vi "Get PI data.vi"() -> ()   [LabVIEW 2017]
panel:
  out "values":T1
  out "error out":errorcluster
  in  "connection ID":refnum<k16>
  in  "error in (no error)":errorcluster
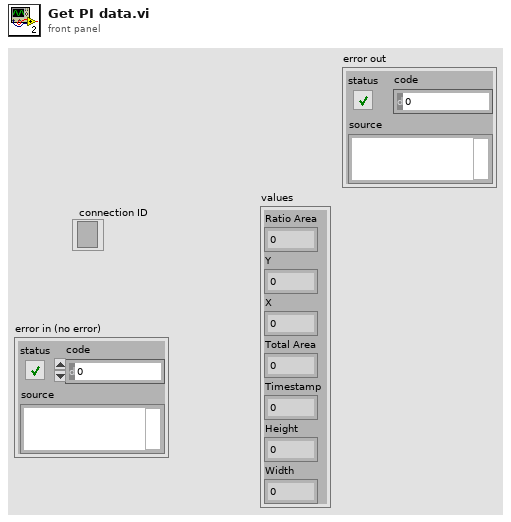
[diagram p1: front panel]
types:
  T1 = cluster{"Ratio Area":dbl, "Y":dbl, "X":dbl, "Total Area":dbl, "Timestamp":ext, "Height":dbl, "Width":dbl}
  T2 = cluster{"RatioArea":dbl, "CenterY":dbl, "CenterX":dbl, "Area":dbl, "Timestamp":ext, "Height":dbl, "Width":dbl}
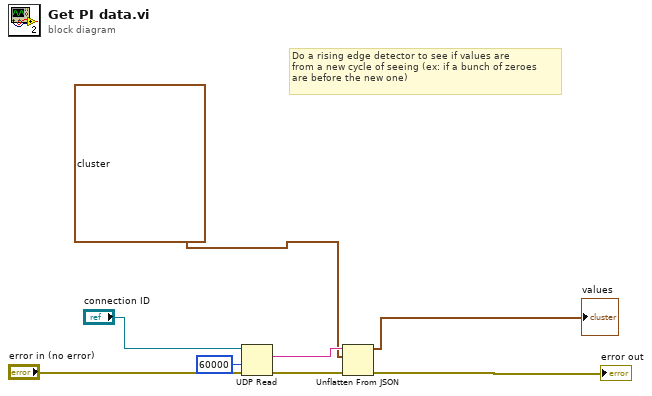
[diagram p0: block diagram]
diagram:
  # "Do a rising edge detector to see if values are \nfrom a new cycle of seeing (ex: if a bunch of zeroes\nare before the new one)"
  n1 = UDP Read(connection ID="connection ID", timeout ms (25000)=60000, 8:"error in (no error)") -> (data out=w6:string, error out=w5:errorcluster)  [unwired: 1 in, 3 out]
  n2 = Unflatten From JSON(JSON string=w6, type and defaults=T2 {"RatioArea"=0.0, "CenterY"=0.0, "CenterX"=0.0, "Area"=0.0, "Timestamp"=0.0, "Height"=0.0, "Width"=0.0}, error in (no error)=w5) -> (value=→"values":T2, error out=→"error out":errorcluster)  [unwired: 4 in]
